vi "ALTER POV.vi"(10 "Boolean":bool, 11 "Array":T4(array[cluster])) -> ()   [LabVIEW 2020]
uses:
  <vilib>/Rock Robotics/WPI/PWM/Servo/WPI_ServoDeviceRef.ctl
  <vilib>/Rock Robotics/SystemInterfaces/DIO/FPGA_DIOPWMChannel.ctl
  <vilib>/Rock Robotics/WPI/PWM/WPI_PWMDeadband.ctl
  <vilib>/Rock Robotics/Network Tables/NT Read Numeric Array.vi
  <vilib>/Rock Robotics/Network Tables/NT Read Boolean Array.vi
  <vilib>/Rock Robotics/Network Tables/NT Read Number.vi
  <vilib>/Rock Robotics/Network Tables/NT Write Number.vi
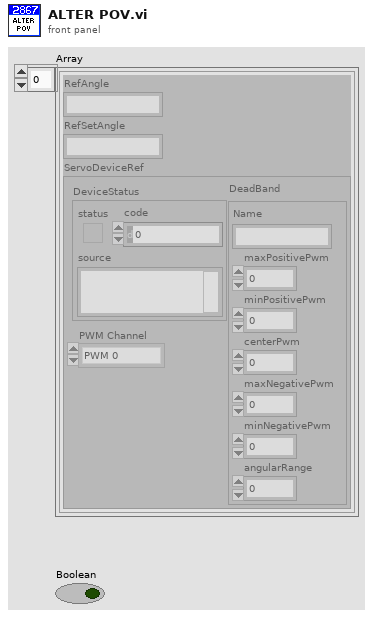
[diagram p1: front panel]
types:
  T1 = typedef "WPI_ServoDeviceRef.ctl" = cluster{"DeviceStatus":errorcluster, "PWM Channel":T2, "DeadBand":T3}
  T2 = typedef "FPGA_DIOPWMChannel.ctl" = enum8{"PWM 0", "PWM 1", "PWM 2", "PWM 3", "PWM 4", "PWM 5", "PWM 6", "PWM 7", "PWM 8", "PWM 9", "PWM MXP 0", "PWM MXP 1", "PWM MXP 2", "PWM MXP 3", "PWM MXP 4", "PWM MXP 5", "PWM MXP 6", "PWM MXP 7", "PWM MXP 8", "PWM MXP 9", "Invalid"}
  T3 = typedef "WPI_PWMDeadband.ctl" = cluster{"Name":string, "maxPositivePwm":i32, "minPositivePwm":i32, "centerPwm":i32, "maxNegativePwm":i32, "minNegativePwm":i32, "angularRange":u16}
  T4 = cluster{"RefAngle":string, "RefSetAngle":string, "ServoDeviceRef":T1}[]
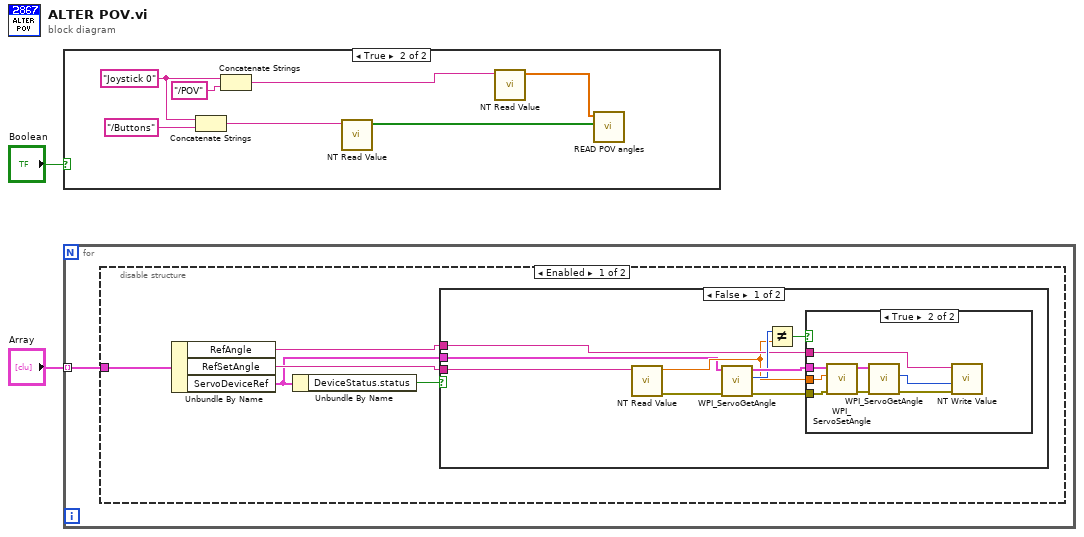
[diagram p0: block diagram]
diagram:
  n1 = case shown="True" "Boolean" {
    frame False {
    }
    frame True {
      w5 = "Joystick 0" ("Name")
      n2 = Concatenate Strings(w5, "/Buttons" ("string")) -> (w4:string)
      n3 = Concatenate Strings(w5, "/POV" ("string")) -> (w9:string)
      n4 = call-poly <vilib>:"NT Read Value.vi"("Name"=w4) -> ("Boolean Array"=w3:bool[])  [unwired: 9 in, 1 out]
      n5 = call-poly <vilib>:"NT Read Value.vi"("Name"=w9) -> ("Numeric Array"=w7:dbl[])  [unwired: 9 in, 1 out]
      n6 = call "READ POV angles.vi"("Buttons"=w3, "POVs"=w7) -> ()  [unwired: 10 in]
    }
  }
  n7 = for {
    tunnel: "Array" -> [w10] mode=indexing
    n8 = disable-structure shown="Enabled" {
      disable-tunnel: w10 -> [w13 _]
      frame Enabled {
        n9 = Unbundle By Name(w13) -> ("RefAngle"=w14:string, "RefSetAngle"=w15:string, "ServoDeviceRef"=w12:T1)
        n10 = Unbundle By Name(w12) -> ("DeviceStatus.status"=w11:bool)
        n11 = case shown="False" w11 {
          tunnel: w15 -> [w21 _]
          tunnel: w14 -> [w20 _]
          tunnel: w12 -> [w17 _]
          frame False {
            n12 = call-poly <vilib>:"NT Read Value.vi"("Name"=w21) -> ("error out"=w16:errorcluster, "Numeric"=w18:dbl)  [unwired: 9 in]
            n13 = call <vilib>:"WPI_ServoGetAngle.vi"("ServoDeviceRef"=w17, "error in (no error)"=w16) -> ("ServoDeviceRef"=w23:T1, "Angle"=w22:u16, "error out"=w24:errorcluster)  [unwired: 6 in]
            n14 = Not Equal?(x=w22, y=w18) -> (x != y?=w19:bool)
            n15 = case shown="True" w19 {
              tunnel: w24 -> [_ w32]
              tunnel: w23 -> [_ w31]
              tunnel: w20 -> [_ w30]
              tunnel: w18 -> [_ w29]
              frame False {
              }
              frame True {
                n16 = call <vilib>:"WPI_ServoSetAngle.vi"("error in (no error)"=w32, "Angle"=w29, "ServoDeviceRef"=w31) -> ("error out"=w27:errorcluster, "ServoDeviceRef"=w28:T1)  [unwired: 7 in]
                n17 = call <vilib>:"WPI_ServoGetAngle.vi"("ServoDeviceRef"=w28, "error in (no error)"=w27) -> ("Angle"=w25:u16, "error out"=w26:errorcluster)  [unwired: 6 in, 1 out]
                n18 = call-poly <vilib>:"NT Write Value.vi"("error in"=w26, "Numeric"=w25, "Name"=w30) -> ()  [unwired: 8 in, 1 out]
              }
            }
          }
          frame True {
          }
        }
      }
      frame Disabled {
      }
    }
  }
